vi "Calibrate Path User Interface.vi"(8 "error in (no error)":errorcluster, 10 "VNA present":bool, 11 "PathControl in":refnum<class "PathControl.lvclass">) -> (0 "error out":errorcluster, 3 "PathControl out":refnum<class "PathControl.lvclass">)   [LabVIEW 2020, in "PathControl.lvclass"]
uses:
  PathControl.lvclass
  Path Cal Enum.ctl
  PathControl.lvclass/PathControl.ctl
  Instruments/Vector Network Analyzer/Vector Network Analyzer.lvclass
panel:
  in  "Paths to calibrate":i32(listbox)=17
  out "Frequency (MHz) | Gain (dB)":T1(array[cluster])
  in  "Load text":bool
  in  "Cancel Button":bool
  in  "Load Manually":bool
  in  "Load Button":bool
  in  "Calibrate VNA":bool
  in  "Done Button":bool
  in  "Run Cal Button":bool
  in  "Deselect all Button":bool
  in  "Select all Button":bool
  out "Current Path Calibration":cluster{dbl[], "Path Loss":dbl[]}(graph)
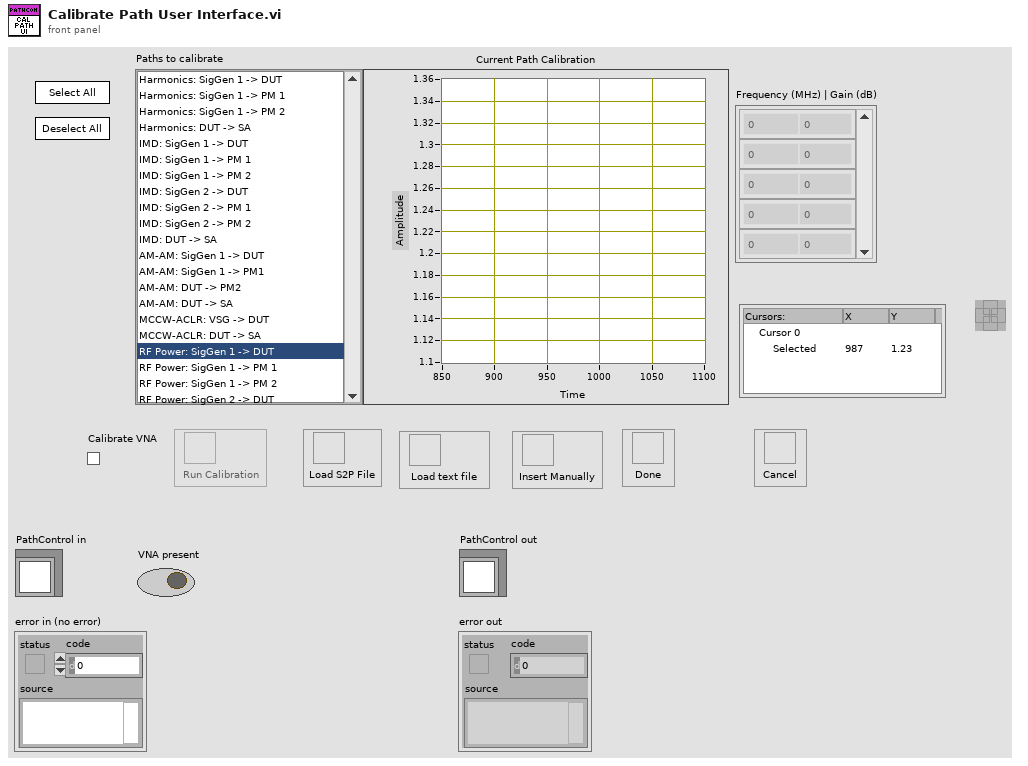
[diagram p1: front panel]
types:
  T1 = cluster{"Frequency (MHz)":dbl, "Gain (dB)":dbl}[]
  T2 = enum8{"Enabled", "Disabled", "Disabled and Grayed Out"}
  T3 = typedef "PathControl.lvclass/Path Cal Enum.ctl" = enum16{"Update Graph", "Update selection", "Calibrate VNA", "Run calibration", "Select All", "Deselect All", "Load S2P File", "Load Manually", "Load Text file", "Done"}
  T4 = cluster{"Path Calibration state machine":T3, variant}
  T5 = cluster{"Name":string, "Path Frequency":dbl[], "Path Loss":dbl[]}
  T6 = cluster{"Name":string, "Path Frequency":dbl[], "Path Loss":dbl[]}[]
  T7 = cluster{"Path Calibration state machine":T3, i32}
  T8 = cluster{"Path Calibration state machine":T3, "Paths to calibrate":i32}
  T9 = cluster{"Path Calibration state machine":T3, "Value":i32}
  T10 = cluster{"Path Calibration state machine":T3, "Done Button":bool}
  T11 = cluster{"Path Calibration state machine":T3, "Variant":variant}
  T12 = cluster{"Path Calibration state machine":T3, "Row":i32}
  T13 = cluster{"Path Calibration state machine":T3, "NewVal":i32}
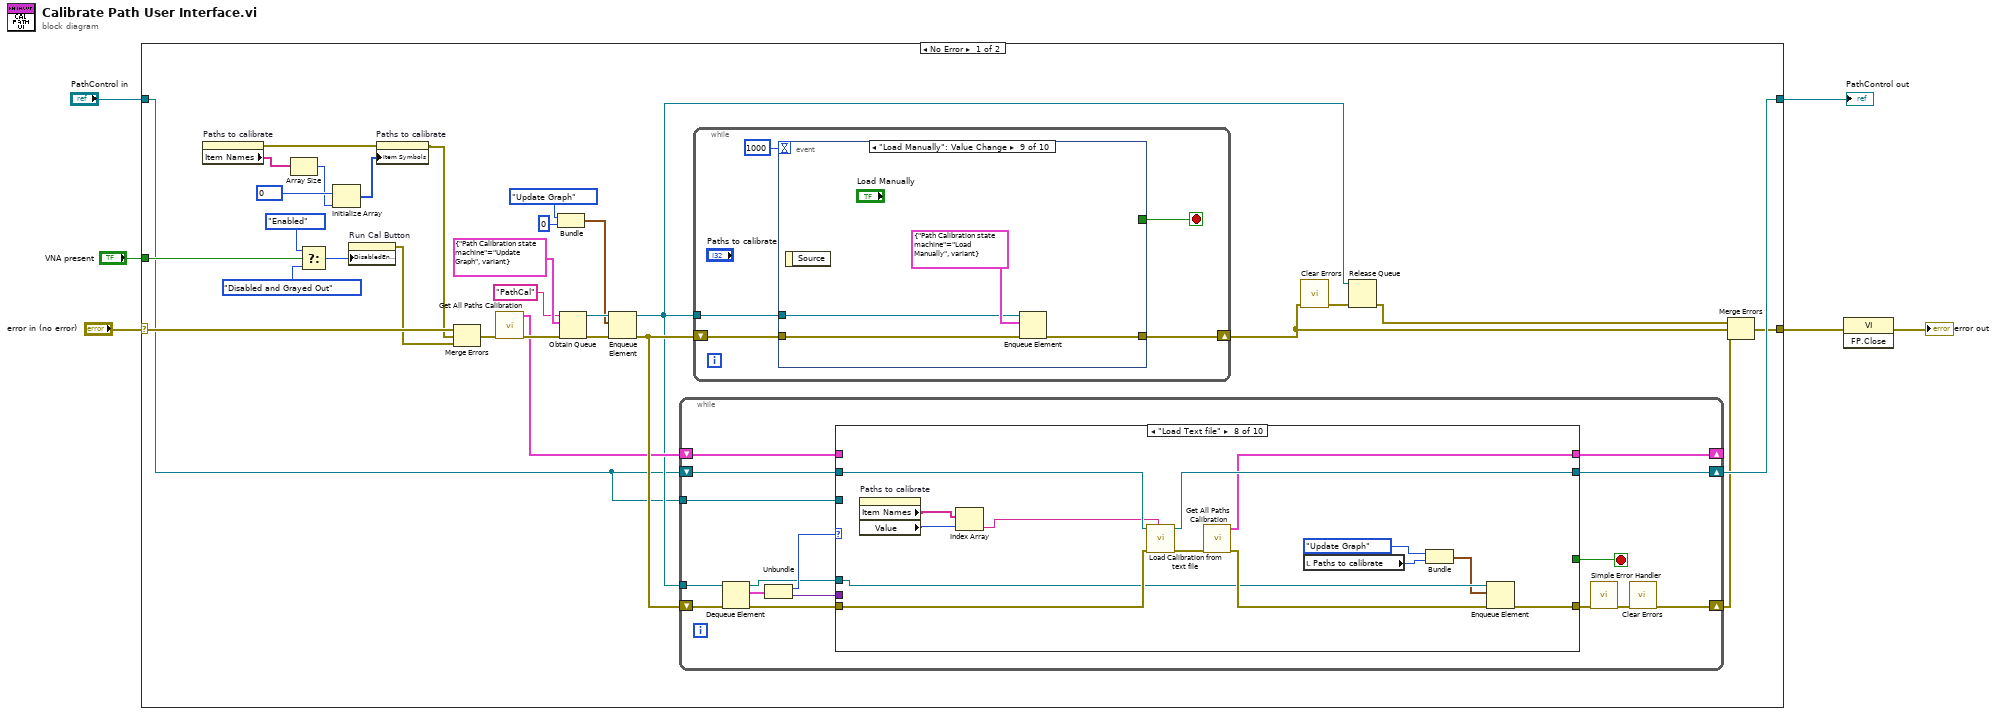
[diagram p0: block diagram]
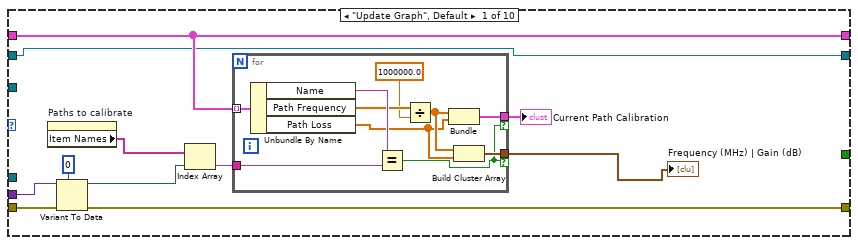
[diagram p2: hidden frame]
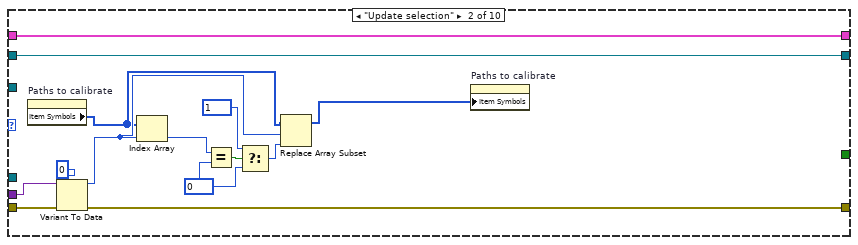
[diagram p3: hidden frame]
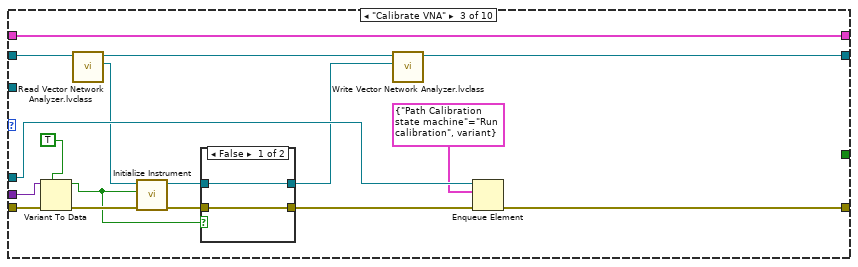
[diagram p4: hidden frame]
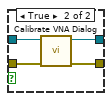
[diagram p5: hidden frame]
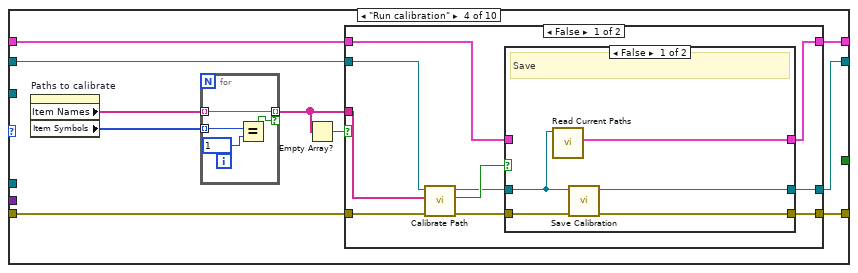
[diagram p6: hidden frame]
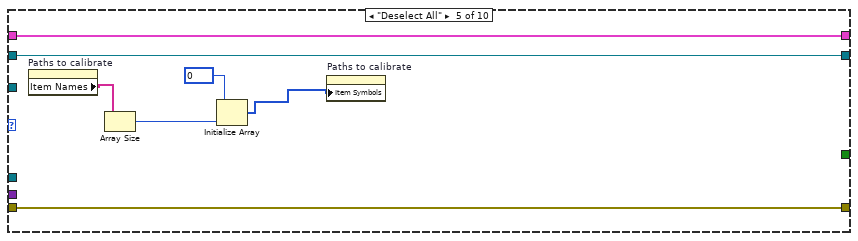
[diagram p9: hidden frame]
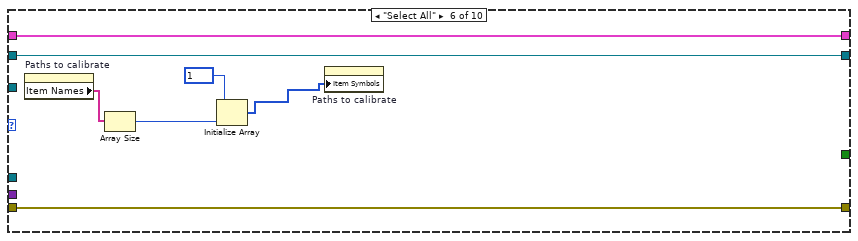
[diagram p10: hidden frame]
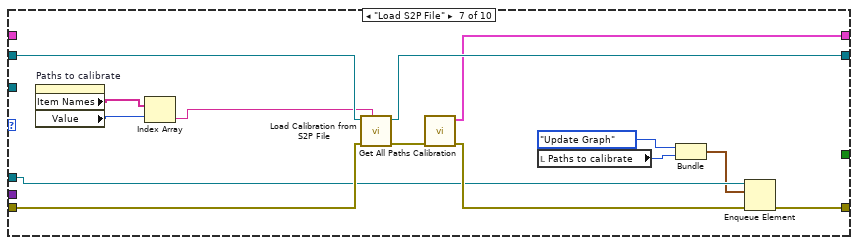
[diagram p11: hidden frame]
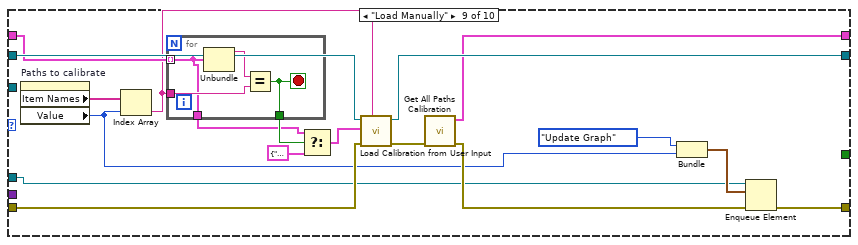
[diagram p12: hidden frame]
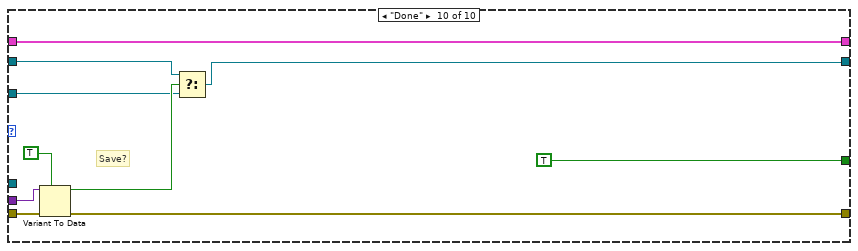
[diagram p13: hidden frame]
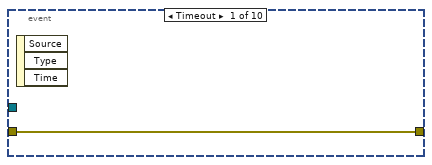
[diagram p14: hidden frame]
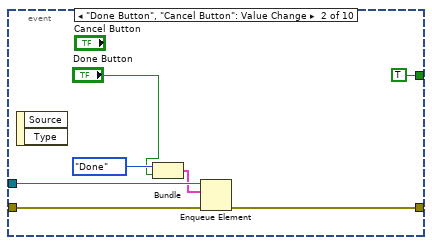
[diagram p15: hidden frame]
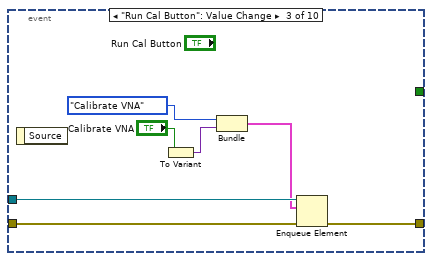
[diagram p16: hidden frame]
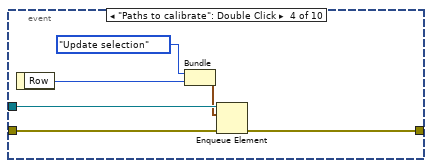
[diagram p17: hidden frame]
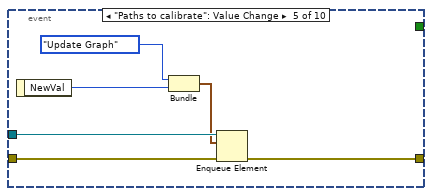
[diagram p18: hidden frame]
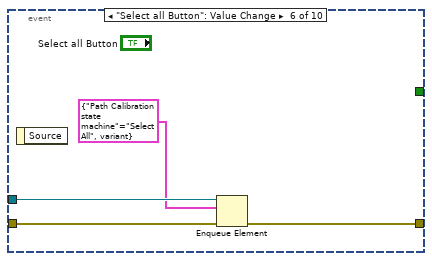
[diagram p19: hidden frame]
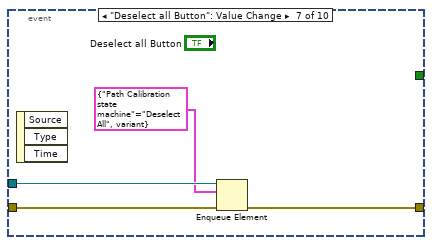
[diagram p20: hidden frame]
diagram:
  n1 = case shown="No Error" "error in (no error)" {
    selector: "error in (no error)" -> [w35 w272]
    tunnel: [w12 w272] -> w2
    tunnel: [w24 w271] -> w4
    tunnel: "PathControl in" -> [w11 w271]
    tunnel: "VNA present" -> [w18 _]
    frame No Error {
      n2 = property on="Paths to calibrate" class="LstBox (strict)"() -> (error out=w7:errorcluster, "Item Names"=w10:string[])  [unwired: 2 in, 1 out]
      n3 = Array Size(array=w10) -> (size(s)=w36:i32)
      n4 = Select(t=T2."Enabled" ("Disabled"), s=w18, f=T2."Disabled and Grayed Out") -> (s? t:f=w20:T2)
      n5 = Initialize Array(0, w36) -> (w8:i32[])
      n6 = property on="Run Cal Button" class="Bool"("DisabledEnum"=w20) -> (error out=w21:errorcluster)  [unwired: 2 in, 1 out]
      n7 = property on="Paths to calibrate" class="LstBox (strict)"(error in=w7, "Item Symbols"=w8) -> (error out=w9:errorcluster)  [unwired: 1 in, 1 out]
      n8 = Merge Errors(w35, w9, w21) -> (w34:errorcluster)
      n9 = call "Get All Paths Calibration.vi"("Error In"=w34) -> ("Error Out"=w33:errorcluster, "All Paths"=w29:T6)  [unwired: 9 in]
      n10 = Bundle("Path Calibration state machine"=Path_Cal_Enum."Update Graph", 0) -> (w25:T7)  [unwired: 1 in]
      n11 = Obtain Queue(name (unnamed)="PathCal", element data type=T4 {"Path Calibration state machine"=enum."Update Graph", variant}, error in (no error)=w33) -> (queue out=w31:refnum<queue>, error out=w32:errorcluster)  [unwired: 2 in, 1 out]
      n12 = Enqueue Element(queue=w31, element=w25, error in (no error)=w32) -> (queue out=w23:refnum<queue>, error out=w30:errorcluster)  [unwired: 1 in, 1 out]
      n13 = while {
        shift-right: [w39] -> w22
        shift-left: w30 -> [w53]
        tunnel: w23 -> [w52]
        shift-right: [w45] -> _
        shift-left: w29 -> [w46]
        shift-right: [w42] -> w24
        shift-left: w11 -> [w43]
        tunnel: w11 -> [w38]
        stop <- w44 stop-if-true
        n14 = Dequeue Element(queue=w52, error in (no error)=w53) -> (queue out=w47:refnum<queue>, element=w51:T4, error out=w48:errorcluster)  [unwired: 1 in, 1 out]
        n15 = Unbundle(w51) -> ("Path Calibration state machine"=w50:T3, w49:variant)
        n16 = case shown="\"Load Text file\"" w50 {
          tunnel: w49 -> [w63 w86 w90 _ _ _ _ _ _ w216]
          tunnel: w48 -> [w64 w87 w93 w120 w150 w157 w171 w184 w202 w215]
          tunnel: w47 -> [_ _ w101 _ _ _ w167 w180 w195 _]
          tunnel: w46 -> [w60 w88 w105 w117 w153 w160 _ _ w194 w218]
          tunnel: [w60 w88 w105 w116 w153 w160 w169 w182 w200 w218] -> w45
          tunnel: [_ _ _ _ _ _ _ _ _ TRUE] -> w44
          tunnel: [w58 w78 w102 w118 w150 w157 w168 w181 w196 w213] -> w41
          tunnel: w43 -> [w57 w77 w104 w121 w149 w156 w173 w186 w204 w212]
          tunnel: [w57 w77 w95 w119 w149 w156 w172 w185 w203 w211] -> w42
          tunnel: w38 -> [_ _ _ _ _ _ _ _ _ w209]
          frame "Update Graph", Default {
            n17 = property on="Paths to calibrate" class="LstBox (strict)"() -> ("Item Names"=w54:string[])  [unwired: 2 in, 2 out]
            n18 = Variant To Data(error in=w64, type=0, Variant=w63) -> (data=w61:i32, error out=w58:errorcluster)
            n19 = Index Array(array=w54, index=w61) -> (element=w59:string)
            n20 = for {
              tunnel: w60 -> [w74] mode=indexing
              tunnel: w59 -> [w72]
              tunnel: [w70] -> w56 if=w65
              tunnel: [w66] -> w55 if=w65
              n21 = Unbundle By Name(w74) -> ("Name"=w73:string, "Path Frequency"=w71:dbl[], "Path Loss"=w67:dbl[])
              n22 = Equal?(x=w73, y=w72) -> (x = y?=w65:bool)
              n23 = Divide(x=w71, y=1000000.0) -> (x/y=w68:dbl[])
              n24 = Bundle(w68, "Path Loss"=w67) -> (w70:cluster{dbl[], "Path Loss":dbl[]})  [unwired: 1 in]
              n25 = Build Cluster Array(w68, w67) -> (w66:cluster{dbl, "Numeric Control":dbl}[])
            }
            "Current Path Calibration" <- w56
            "Frequency (MHz) | Gain (dB)" <- w55
          }
          frame "Update selection" {
            w81 = 0
            n26 = property on="Paths to calibrate" class="LstBox (strict)"() -> ("Item Symbols"=w76:i32[])  [unwired: 2 in, 2 out]
            n27 = Variant To Data(error in=w87, type=0, Variant=w86) -> (data=w80:i32, error out=w78:errorcluster)
            n28 = Index Array(array=w76, index=w80) -> (element=w84:i32)
            n29 = Equal?(x=w84, y=w81) -> (x = y?=w83:bool)
            n30 = Select(t=1, s=w83, f=w81) -> (s? t:f=w79:i32)
            n31 = Replace Array Subset(array=w76, new element=w79, index=w80) -> (w75:i32[])
            n32 = property on="Paths to calibrate" class="LstBox (strict)"("Item Symbols"=w75) -> ()  [unwired: 2 in, 2 out]
          }
          frame "Calibrate VNA" {
            n33 = Variant To Data(error in=w93, type=TRUE ("Reset"), Variant=w90) -> (data=w89:bool, error out=w92:errorcluster)
            n34 = call "Read Vector Network Analyzer.lvclass.vi"("PathControl in"=w104) -> ("Vector Network Analyzer.lvclass"=w97:refnum<class "Vector Network Analyzer.lvclass">, "PathControl out"=w96:refnum<class "PathControl.lvclass">)  [unwired: 9 in]
            n35 = call-dynamic "Initialize Instrument.vi"("error in (no error)"=w92, "Reset"=w89, "Instrument in"=w97) -> ("error out"=w99:errorcluster, "Instrument out"=w98:refnum<class "Vector Network Analyzer.lvclass">)  [unwired: 7 in]
            n36 = case shown="False" w89 {
              tunnel: [w107 w111] -> w103
              tunnel: w99 -> [w107 w110]
              tunnel: w98 -> [w106 w109]
              tunnel: [w106 w108] -> w94
              frame False {
              }
              frame True {
                n37 = call "Calibrate VNA Dialog.vi"("error in (no error)"=w110, "Vector Network Analyzer in"=w109) -> ("error out"=w111:errorcluster, "Vector Network Analyzer out"=w108:refnum<class "Vector Network Analyzer.lvclass">)  [unwired: 8 in]
              }
            }
            n38 = call "Write Vector Network Analyzer.lvclass.vi"("Vector Network Analyzer.lvclass"=w94, "PathControl in"=w96) -> ("PathControl out"=w95:refnum<class "PathControl.lvclass">)  [unwired: 9 in]
            n39 = Enqueue Element(queue=w101, element=T4 {"Path Calibration state machine"=enum."Run calibration", variant}, error in (no error)=w103) -> (error out=w102:errorcluster)  [unwired: 1 in, 2 out]
          }
          frame "Run calibration" {
            n40 = property on="Paths to calibrate" class="LstBox (strict)"() -> ("Item Names"=w113:string[], "Item Symbols"=w112:i32[])  [unwired: 2 in, 2 out]
            n41 = for {
              tunnel: w113 -> [w144] mode=indexing
              tunnel: w112 -> [w146] mode=indexing
              tunnel: [w144] -> w115 mode=indexing if=w143
              n42 = Equal?(x=w146, y=1) -> (x = y?=w143:bool)
            }
            n43 = Empty Array?(array=w115) -> (empty?=w114:bool)
            n44 = case shown="False" w114 {
              tunnel: w121 -> [w131 w141]
              tunnel: w120 -> [w130 w142]
              tunnel: [w126 w141] -> w119
              tunnel: [w125 w142] -> w118
              tunnel: w117 -> [w124 w140]
              tunnel: [w123 w140] -> w116
              tunnel: w115 -> [w122 _]
              frame False {
                n45 = call "Calibrate Path.vi"("error in (no error)"=w130, "Names"=w122, "PathControl in"=w131) -> ("error out"=w127:errorcluster, "Canceled?"=w129:bool, "PathControl out"=w128:refnum<class "PathControl.lvclass">)  [unwired: 6 in]
                n46 = case shown="False" w129 {
                  tunnel: w128 -> [w133 w138]
                  tunnel: w127 -> [w136 w139]
                  tunnel: [w135 w138] -> w126
                  tunnel: [w134 w139] -> w125
                  tunnel: w124 -> [_ w137]
                  tunnel: [w132 w137] -> w123
                  frame False {
                    # "Save"
                    n47 = call "Read Current Paths.vi"("PathControl in"=w133) -> ("Current Paths"=w132:T6)  [unwired: 9 in, 1 out]
                    n48 = call "Save Calibration.vi"("error in (no error)"=w136, "PathControl in"=w133) -> ("error out"=w134:errorcluster, "PathControl out"=w135:refnum<class "PathControl.lvclass">)  [unwired: 8 in]
                  }
                  frame True {
                    # "Don't save"
                  }
                }
              }
              frame True {
              }
            }
          }
          frame "Deselect All" {
            n49 = property on="Paths to calibrate" class="LstBox (strict)"() -> ("Item Names"=w148:string[])  [unwired: 2 in, 2 out]
            n50 = Array Size(array=w148) -> (size(s)=w152:i32)
            n51 = Initialize Array(0, w152) -> (w147:i32[])
            n52 = property on="Paths to calibrate" class="LstBox (strict)"("Item Symbols"=w147) -> ()  [unwired: 2 in, 2 out]
          }
          frame "Select All" {
            n53 = property on="Paths to calibrate" class="LstBox (strict)"() -> ("Item Names"=w155:string[])  [unwired: 2 in, 2 out]
            n54 = Array Size(array=w155) -> (size(s)=w159:i32)
            n55 = Initialize Array(1, w159) -> (w154:i32[])
            n56 = property on="Paths to calibrate" class="LstBox (strict)"("Item Symbols"=w154) -> ()  [unwired: 2 in, 2 out]
          }
          frame "Load S2P File" {
            n57 = property on="Paths to calibrate" class="LstBox (strict)"() -> ("Item Names"=w162:string[], "Value"=w161:i32)  [unwired: 2 in, 2 out]
            n58 = Index Array(array=w162, index=w161) -> (element=w163:string)
            n59 = call "Load Calibration from S2P File.vi"("path"=w163, "error in (no error)"=w171, "PathControl in"=w173) -> ("error out"=w170:errorcluster, "PathControl out"=w172:refnum<class "PathControl.lvclass">)  [unwired: 7 in]
            n60 = call "Get All Paths Calibration.vi"("Error In"=w170) -> ("Error Out"=w168:errorcluster, "All Paths"=w169:T6)  [unwired: 9 in]
            n61 = local read "Paths to calibrate"() -> (w165:i32)
            n62 = Bundle("Path Calibration state machine"=Path_Cal_Enum."Update Graph", "Paths to calibrate"=w165) -> (w164:T8)  [unwired: 1 in]
            n63 = Enqueue Element(queue=w167, element=w164, error in (no error)=w168) -> ()  [unwired: 1 in, 3 out]
          }
          frame "Load Text file" {
            n64 = property on="Paths to calibrate" class="LstBox (strict)"() -> ("Item Names"=w175:string[], "Value"=w174:i32)  [unwired: 2 in, 2 out]
            n65 = Index Array(array=w175, index=w174) -> (element=w176:string)
            n66 = call "Load Calibration from text file.vi"("path"=w176, "error in (no error)"=w184, "PathControl in"=w186) -> ("error out"=w183:errorcluster, "PathControl out"=w185:refnum<class "PathControl.lvclass">)  [unwired: 7 in]
            n67 = call "Get All Paths Calibration.vi"("Error In"=w183) -> ("Error Out"=w181:errorcluster, "All Paths"=w182:T6)  [unwired: 9 in]
            n68 = local read "Paths to calibrate"() -> (w178:i32)
            n69 = Bundle("Path Calibration state machine"=Path_Cal_Enum."Update Graph", "Paths to calibrate"=w178) -> (w177:T8)  [unwired: 1 in]
            n70 = Enqueue Element(queue=w180, element=w177, error in (no error)=w181) -> ()  [unwired: 1 in, 3 out]
          }
          frame "Load Manually" {
            n71 = property on="Paths to calibrate" class="LstBox (strict)"() -> ("Item Names"=w188:string[], "Value"=w187:i32)  [unwired: 2 in, 2 out]
            n72 = Index Array(array=w188, index=w187) -> (element=w189:string)
            n73 = for {
              tunnel: w194 -> [w206] mode=indexing
              tunnel: w189 -> [w207]
              tunnel: [w206] -> w192
              tunnel: [w205] -> w193
              stop <- w205 stop-if-true
              n74 = Unbundle(w206) -> ("Name"=w208:string)  [unwired: 2 out]
              n75 = Equal?(x=w208, y=w207) -> (x = y?=w205:bool)
            }
            n76 = Select(t=w192, s=w193, f=T5 {"Name"="", "Path Frequency"=[], "Path Loss"=[]}) -> (s? t:f=w191:T5)
            n77 = call "Load Calibration from User Input.vi"("path"=w189, "error in (no error)"=w202, "Old values"=w191, "PathControl in"=w204) -> ("error out"=w201:errorcluster, "PathControl out"=w203:refnum<class "PathControl.lvclass">)  [unwired: 6 in]
            n78 = call "Get All Paths Calibration.vi"("Error In"=w201) -> ("Error Out"=w197:errorcluster, "All Paths"=w200:T6)  [unwired: 9 in]
            n79 = Bundle("Path Calibration state machine"=Path_Cal_Enum."Update Graph", "Value"=w187) -> (w199:T9)  [unwired: 1 in]
            n80 = Enqueue Element(queue=w195, element=w199, error in (no error)=w197) -> (error out=w196:errorcluster)  [unwired: 1 in, 2 out]
          }
          frame "Done" {
            # "Save?"
            n81 = Variant To Data(error in=w215, type=TRUE, Variant=w216) -> (data=w210:bool, error out=w213:errorcluster)
            n82 = Select(t=w212, s=w210, f=w209) -> (s? t:f=w211:refnum<class "PathControl.lvclass">)
          }
        }
        n83 = call <vilib>:"Simple Error Handler.vi"("error in (no error)"=w41) -> ("error out"=w40:errorcluster)  [unwired: 4 in, 4 out]
        n84 = call <vilib>:"Clear Errors.vi"("error in (no error)"=w40) -> ("error out"=w39:errorcluster)  [unwired: 5 in, 1 out]
      }
      n85 = while {
        shift-right: [w221] -> w15
        shift-left: w30 -> [w223]
        tunnel: w23 -> [w222]
        stop <- w220 stop-if-true
        n86 = event shown="[8] \"Load Manually\": Value Change" {
          selector: _ -> [_ _ _ _ _ _ _ _ _ _]
          dyn-events: _ -> [_ _ _ _ _ _ _ _ _ _]
          timeout: 1000 -> [_ _ _ _ _ _ _ _ _ _]
          tunnel: w223 -> [w224 w231 w237 w244 w250 w253 w256 w260 w264 w268]
          tunnel: w222 -> [_ w230 w236 w243 w249 w252 w257 w261 w265 w269]
          tunnel: [w224 w229 w238 w242 w246 w254 w258 w259 w263 w267] -> w221
          tunnel: [_ TRUE ("Done Button") _ _ _ _ _ _ _ _] -> w220
          event Timeout {
            n87 = event-data() -> ()  [unwired: 1 in, 3 out]
          }
          event "Done Button", "Cancel Button": Value Change {
            n88 = event-data() -> ()  [unwired: 1 in, 2 out]
            n89 = Bundle("Path Calibration state machine"=Path_Cal_Enum."Done", "Done Button"="Done Button") -> (w228:T10)  [unwired: 1 in]
            n90 = Enqueue Element(queue=w230, element=w228, error in (no error)=w231) -> (error out=w229:errorcluster)  [unwired: 1 in, 2 out]
          }
          event "Run Cal Button": Value Change {
            n91 = event-data() -> ()  [unwired: 1 in, 1 out]
            n92 = To Variant(anything="Calibrate VNA") -> (Variant=w233:variant)
            n93 = Bundle("Path Calibration state machine"=Path_Cal_Enum."Calibrate VNA", "Variant"=w233) -> (w232:T11)  [unwired: 1 in]
            n94 = Enqueue Element(queue=w236, element=w232, error in (no error)=w237) -> (error out=w238:errorcluster)  [unwired: 1 in, 2 out]
          }
          event "Paths to calibrate": Double Click {
            n95 = event-data() -> ("Row"=w240:i32)  [unwired: 1 in]
            n96 = Bundle("Path Calibration state machine"=Path_Cal_Enum."Update selection", "Row"=w240) -> (w239:T12)  [unwired: 1 in]
            n97 = Enqueue Element(queue=w243, element=w239, error in (no error)=w244) -> (error out=w242:errorcluster)  [unwired: 1 in, 2 out]
          }
          event "Paths to calibrate": Value Change {
            n98 = event-data() -> ("NewVal"=w245:i32)  [unwired: 1 in]
            n99 = Bundle("Path Calibration state machine"=Path_Cal_Enum."Update Graph", "NewVal"=w245) -> (w247:T13)  [unwired: 1 in]
            n100 = Enqueue Element(queue=w249, element=w247, error in (no error)=w250) -> (error out=w246:errorcluster)  [unwired: 1 in, 2 out]
          }
          event "Select all Button": Value Change {
            n101 = event-data() -> ()  [unwired: 1 in, 1 out]
            n102 = Enqueue Element(queue=w252, element=T4 {"Path Calibration state machine"=enum."Select All", variant}, error in (no error)=w253) -> (error out=w254:errorcluster)  [unwired: 1 in, 2 out]
          }
          event "Deselect all Button": Value Change {
            n103 = event-data() -> ()  [unwired: 1 in, 3 out]
            n104 = Enqueue Element(queue=w257, element=T4 {"Path Calibration state machine"=enum."Deselect All", variant}, error in (no error)=w256) -> (error out=w258:errorcluster)  [unwired: 1 in, 2 out]
          }
          event "Load Button": Value Change {
            n105 = event-data() -> ()  [unwired: 1 in, 1 out]
            n106 = Enqueue Element(queue=w261, element=T4 {"Path Calibration state machine"=enum."Load S2P File", variant}, error in (no error)=w260) -> (error out=w259:errorcluster)  [unwired: 1 in, 2 out]
          }
          event "Load Manually": Value Change {
            n107 = event-data() -> ()  [unwired: 1 in, 1 out]
            n108 = Enqueue Element(queue=w265, element=T4 {"Path Calibration state machine"=enum."Load Manually", variant}, error in (no error)=w264) -> (error out=w263:errorcluster)  [unwired: 1 in, 2 out]
          }
          event "Load text": Value Change {
            n109 = event-data() -> ()  [unwired: 1 in, 1 out]
            n110 = Enqueue Element(queue=w269, element=T4 {"Path Calibration state machine"=enum."Load Text file", variant}, error in (no error)=w268) -> (error out=w267:errorcluster)  [unwired: 1 in, 2 out]
          }
        }
      }
      n111 = call <vilib>:"Clear Errors.vi"("error in (no error)"=w15) -> ("error out"=w14:errorcluster)  [unwired: 5 in, 1 out]
      n112 = Release Queue(queue=w23, error in (no error)=w14) -> (error out=w13:errorcluster)  [unwired: 1 in, 2 out]
      n113 = Merge Errors(w13, w15, w22) -> (w12:errorcluster)
    }
    frame Error {
    }
  }
  "PathControl out" <- w4
  n114 = invoke class="VI" method="FP.Close"(error in=w2) -> (error out=→"error out":errorcluster)  [unwired: 2 in, 2 out]
